vi "Sweep Type.vi"(5 "Sweep Type (F:Linear)":bool, 7 "Sweep Direction (F:Down)":bool, 8 "error in (no error)":errorcluster, 9 "Manual Point Value (0.0)":dbl format="%.3f", 10 "Sweep Mode (0:Repeat)":u32(ring) items=["Repeat", "Single", "Manual Point Mode"], 11 "VISA resource name":refnum<visa-resource-name>) -> (0 "error out":errorcluster, 3 "VISA resource name out":refnum<visa-resource-name>)   [LabVIEW 2011, in "Agilent 4194.lvlib"]
doc: "This function sets the sweep type."
uses:
  <instrlib>/Agilent 4194/Agilent 4194.lvlib
panel:
  # "Up"
  # "Logarithmic"
  # "Down"
  # "Linear"
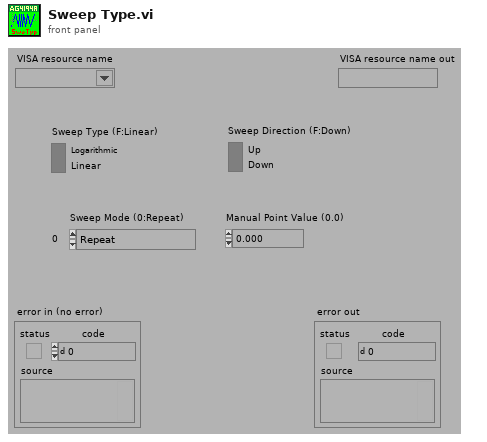
[diagram p1: front panel]
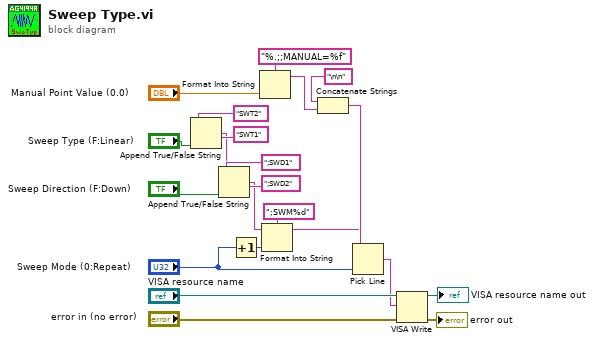
[diagram p0: block diagram]
diagram:
  n1 = Append True/False String(1:"Sweep Type (F:Linear)", 2:"SWT1", 3:"SWT2") -> (0:w10:string)  [unwired: 1 in]
  n2 = Append True/False String(1:"Sweep Direction (F:Down)", 2:";SWD2", 3:";SWD1", 4:w10) -> (0:w7:string)
  n3 = Increment(x="Sweep Mode (0:Repeat)") -> (x+1=w9:u32)
  n4 = Format Into String(format string="%.;;MANUAL=%f", "Manual Point Value (0.0)") -> (resulting string=w2:string)  [unwired: 2 in, 1 out]
  n5 = Format Into String(format string=";SWM%d", initial string=w7, w9) -> (resulting string=w5:string)  [unwired: 1 in, 1 out]
  n6 = Concatenate Strings("\n\n", w2) -> (w6:string)
  n7 = Pick Line(string ("")=w5, multi-line string=w6, line index="Sweep Mode (0:Repeat)") -> (output string=w4:string)
  n8 = VISA Write(VISA resource name="VISA resource name", write buffer=w4, error in (no error)="error in (no error)") -> (VISA resource name out=→"VISA resource name out":refnum<visa-resource-name>, error out=→"error out":errorcluster)  [unwired: 1 out]
